vi "oa_Tachless Speed Profile Generator Popup.vi"(0 "scaled signal [EU]":waveform(dbl)={"t0"=timestamp(0 s since 1904-01-01), "dt"=0.0, "Y"=[]}) -> (3 "effective bandwidth":T3={"bandwidth value"=0.5, "bandwidth unit"=enum."Order"} {"bandwidth value" min=0.0 format="%.2f"}, 4 "dup scaled signal [EU]":waveform(dbl), 8 "speed profile":T4 {"speed [RPM]" format="%.2f"; "time [s]" format="%.2f"}, 10 "orders list":dbl[](array[numeric]) format="%.2f", 14 "window info":T5={"window type"=62, "window length"=2048} {"window type" items=["None"=0, "Hanning"=1, "Hamming"=2, "Blackman-Harris"=3, "Exact Blackman"=4, "Blackman"=5, "Flat Top"=6, "4 Term B-Harris"=7, "7 Term B-Harris"=8, "Low Sidelobe"=9, "Gaussian"=62]; "window length" min=0}, 15 "error out":errorcluster)   [LabVIEW 2017, in "SoundVib_Tachless.lvlib"]
doc: "Interactively generates speed profile from the vibration signal without tachometer signal."
uses:
  <vilib>/addons/Sound and Vibration/Order Analysis/Tachless/SoundVib_Tachless.lvlib
  <vilib>/addons/Sound and Vibration/Order Analysis/Ref Gabor Order Tracking/window information.ctl
  <vilib>/addons/Sound and Vibration/Order Analysis/Tach Process/SubVIs/speed profile.ctl
  <vilib>/addons/Sound and Vibration/Order Analysis/Ref Gabor Order Tracking/Mask Bandwidth.ctl
  <vilib>/Utility/miscctls.llb/LVPoint32TypeDef.ctl
  <vilib>/addons/Sound and Vibration/Order Analysis/Tachless/SubVIs/OAT Tachless Globa Settings.vi
  <vilib>/addons/Sound and Vibration/Order Analysis/Ref Gabor Order Tracking/Get Freq-Time Spectral Map (DBL).vi
  <vilib>/addons/Sound and Vibration/Order Analysis/_OAT State Machine/OAT State Machine Generate Event for Numeric.vi
  <vilib>/addons/Sound and Vibration/Order Analysis/Gabor Order Tracking/SoundVib_Gabor.lvlib
  <vilib>/addons/Sound and Vibration/Order Analysis/Tach Process/SoundVib_TachProcess.lvlib
panel:
  out "MouseButton":u16
  in  "symbols":i32[](array[numeric])=[8, 8, 0, 9, 9]
  in  "Items List":string[](array[string])=["Add Control Point", "Connect", "-", "Remove Control Point", "Break"]
  out "MouseCoords":T1
  out "Cursor Position":cluster{"Cursor X":dbl, "Cursor Y":dbl}
  out "XY Max Range":T2 {"YScale.Range"."Start" format="%.2f"; "YScale.Range"."Minor Incr" format="%.2f"; "YScale.Range"."Increment" format="%.2f"; "YScale.Range"."Maximum" format="%.2f"; "YScale.Range"."Minimum" format="%.2f"; "XScale.Range"."Start" format="%.2f"; "XScale.Range"."Minor Incr" format="%.2f"; "XScale.Range"."Increment" format="%.2f"; "XScale.Range"."Maximum" format="%.2f"; "XScale.Range"."Minimum" format="%.2f"}
  out "sample rate":dbl
  in  "Next":bool
  in  "Prev":bool
  in  "Cancel":bool
  in  "Update Cursor":bool
  in  "Refined Trace Color":u32(colorbox) caption="Color"
  out "new plot":bool=TRUE
  in  "Highlighted Trace Color":u32(colorbox)
  in  "Editing Trace Color":u32(colorbox)
  in  "Mask Color":u32(colorbox)
  out "ignore cursor":bool=TRUE
  in  "Popup Menu":i32(listbox)
  in  "Pop Pos":cluster{i32, i32}
  in  "chkpoint color":u32(colorbox)=16383857
  out "Tracks":cluster{"X":dbl[], "Y":dbl[]}[](graph)
  out "S&V plot":dbl[](graph)
  out "Time-Frequency Plot":dbl[][](graph)
  in  "Pos of Plot Area":bool
  in  "Tab Control":enum32{"Edit", "Refine"}(tab)
  in  "Window Length":T6(ring)=enum."512"
  in  "Current Order":dbl=1.0 format="%.2f"
  in  "Del Order":bool
  in  "Add Order":bool
  in  "Order":dbl=1.0 format="%.2f"
  in  "Reference Orders":i32[](listbox)
  in  "Show Mask":bool
  in  "Refine":bool
  in  "Bandwidth":cluster{"Mask Width":dbl, "unit":u16} {"unit" items=["Order", "Hz"]; "Mask Width" min=0.0 step=0.01 scale=0.001..1.0 scale format="%.2p"}
  # "Data"
  # "State"
  # "Mouse Popup Menu"
  # "Step 1/2 (Edit Profile)"
  # "Setting for Time-Frequency Chart"
  # "Setting for the Control Points"
  # "Tips"
  # "In this step, you should mark one certain order on the Time-Frequency Plot with control points. You can change the Window Length to make the plot clear, and edit the control points by right clicking on it. You should set the Current Order to the one you mark before going to the next step."
  # "Step 2/2 (Refine)"
  # "Setting for Refining"
  # "narrow"
  # "wide"
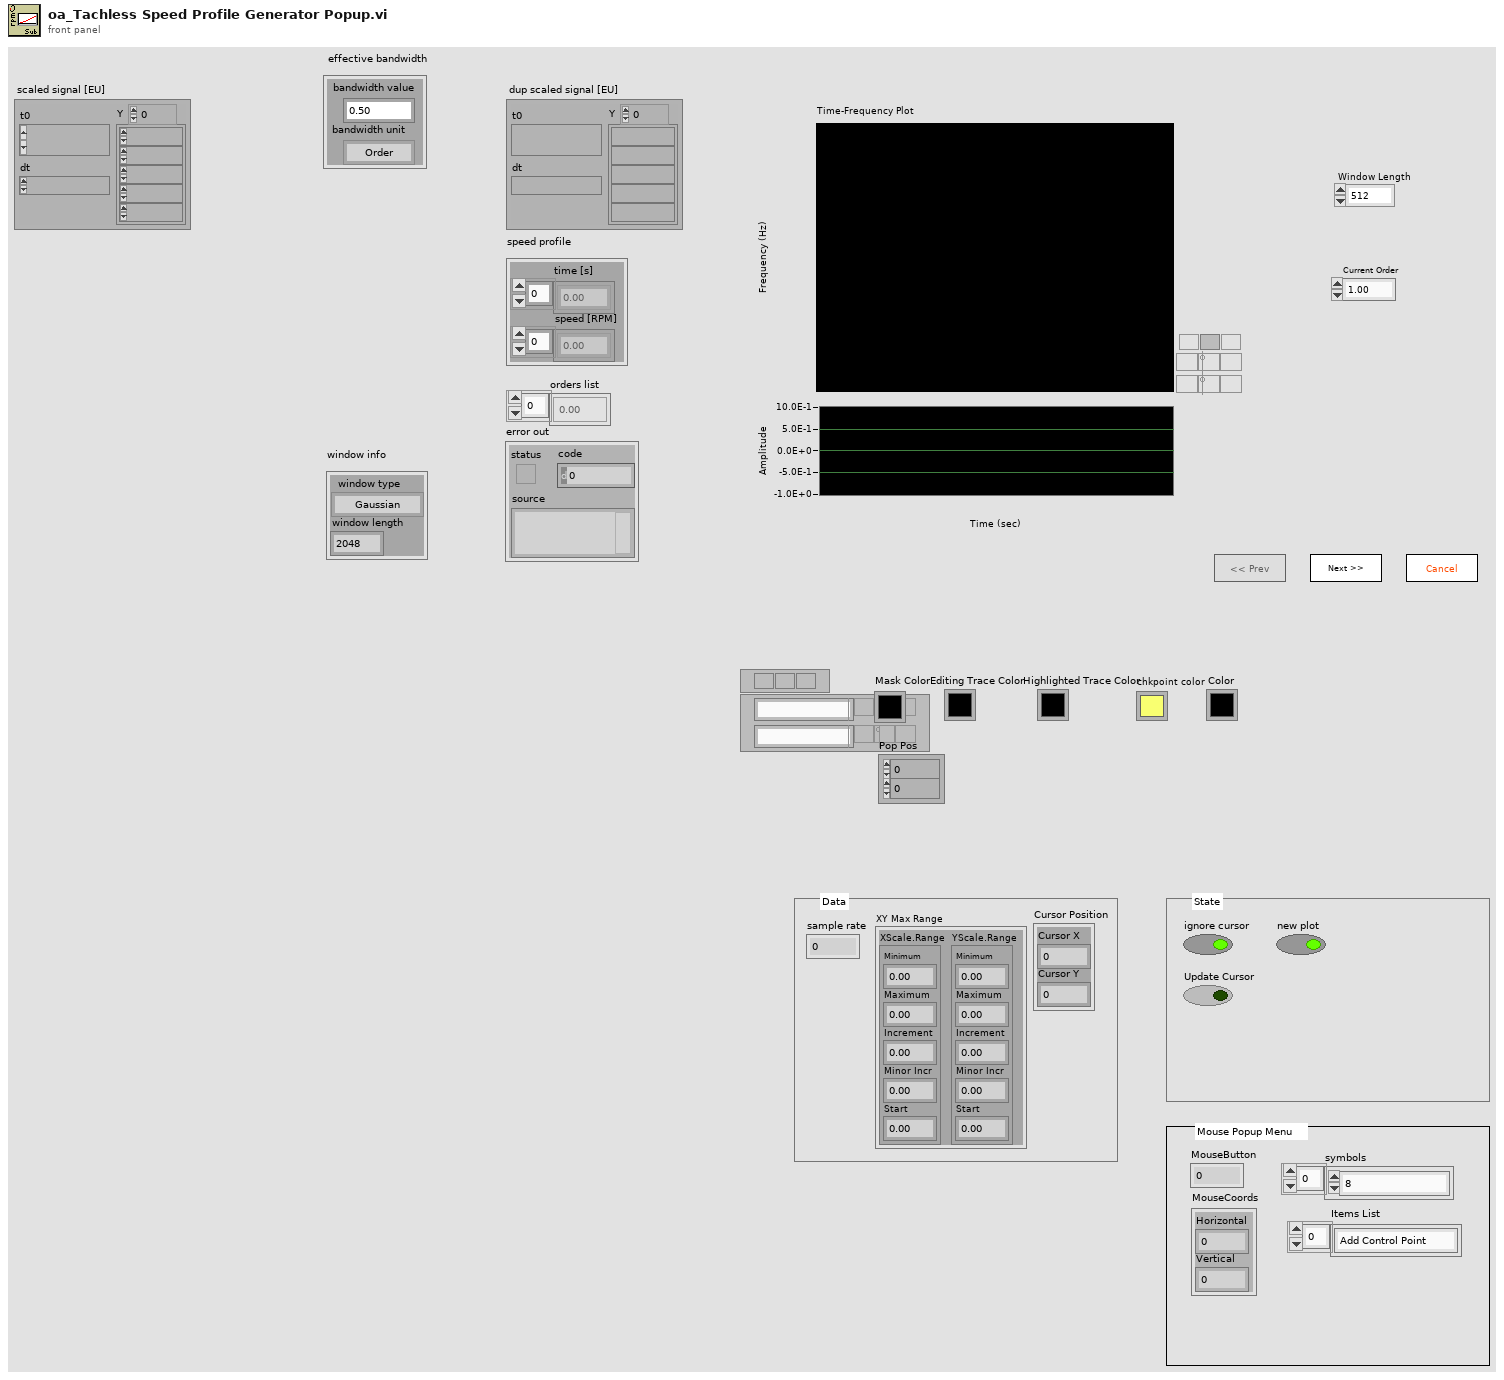
[diagram p1: front panel]
types:
  T1 = typedef "LVPoint32TypeDef.ctl" = cluster{"Horizontal":i32, "Vertical":i32}
  T2 = cluster{"XScale.Range":cluster{"Minimum":dbl, "Maximum":dbl, "Increment":dbl, "Minor Incr":dbl, "Start":dbl}, "YScale.Range":cluster{"Minimum":dbl, "Maximum":dbl, "Increment":dbl, "Minor Incr":dbl, "Start":dbl}}
  T3 = typedef "SoundVib_Gabor.lvlib/Mask Bandwidth.ctl" = cluster{"bandwidth value":dbl, "bandwidth unit":enum16{"Order", "Hz"}}
  T4 = typedef "SoundVib_TachProcess.lvlib/speed profile.ctl" = cluster{"time [s]":dbl[], "speed [RPM]":dbl[]}
  T5 = typedef "SoundVib_Gabor.lvlib/window information.ctl" = cluster{"window type":u32, "window length":i32}
  T6 = enum16{"256", "512", "1024", "2048", "4096", "8192", "16384", "32768"}
  T7 = typedef "LVPositionTypeDef.ctl" = cluster{"Left":i32, "Top":i32}
  T8 = typedef "LVBoundsTypeDef.ctl" = cluster{"Width":u32, "Height":u32}
  T9 = cluster{"Name":string, "Color":u32, "Style":u8, "Point Style":u8, "Name Visible":bool, "Allow Drag":bool, "Lock Style":u32, "Plot":u32, "Index":i32, "Position":cluster{"X":dbl, "Y":dbl}}[]
  T10 = typedef "LVPointDoubleTypeDef.ctl" = cluster{"Cursor X":dbl, "Cursor Y":dbl}
  T11 = typedef "LVRangeTypeDef.ctl" = cluster{"Minimum":dbl, "Maximum":dbl, "Increment":dbl, "Minor Increment":dbl, "Start":dbl}
  T12 = typedef "SoundVib_Gabor.lvlib/GT RefNum.ctl" = refnum<k1>
  T13 = cluster{"Cursor.Cursor X":dbl, "Cursor.Cursor X":dbl}
  T14 = cluster{"Name":string, "Color":u32, "Hair Style":u8, "Point Style":u8, "Name Visible":bool, "Trackable":bool, "Lock Style":u32, "Plot Number":u32, "Marker Index":i32, "Location":cluster{"X":dbl, "Y":dbl}}[]
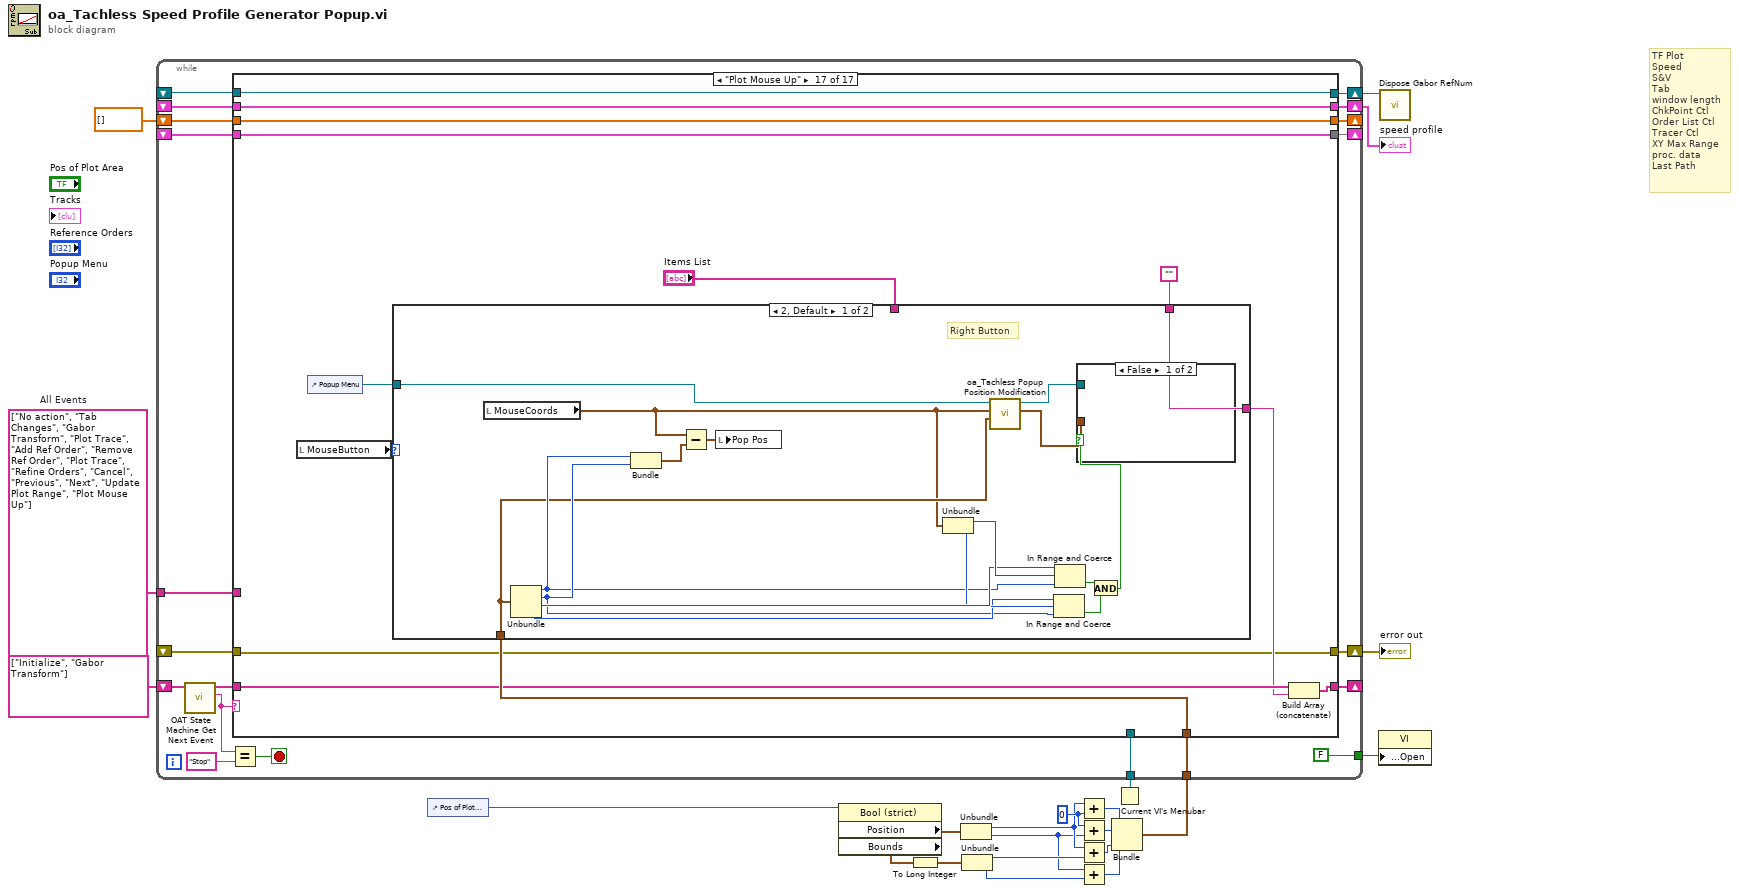
[diagram p0: block diagram]
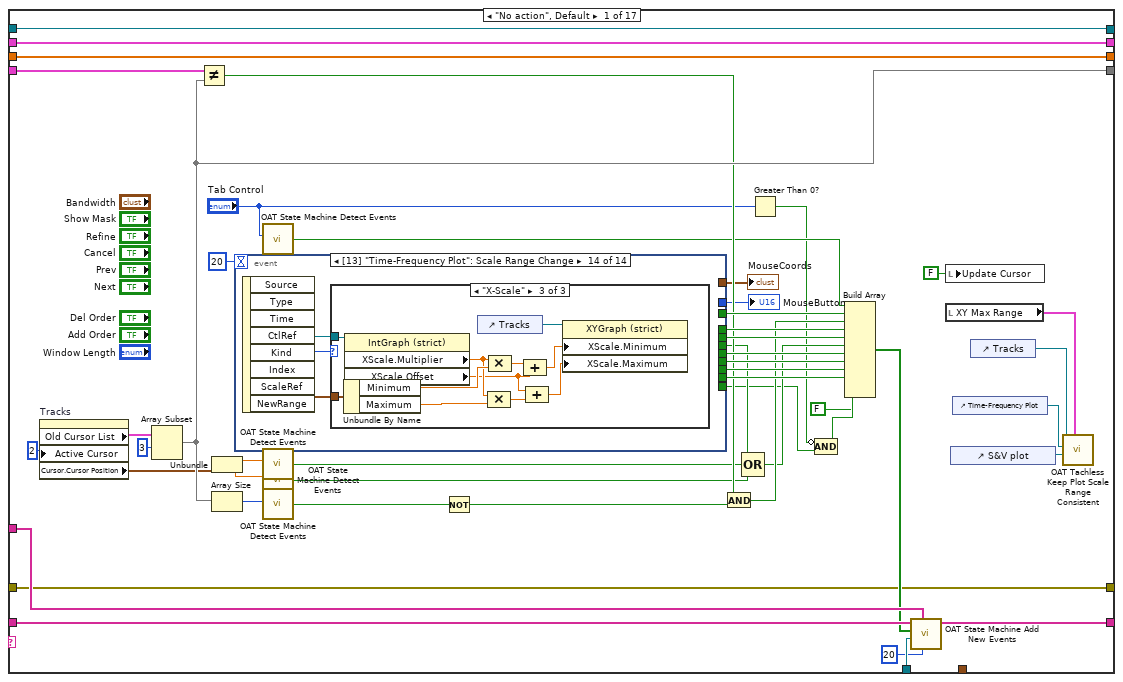
[diagram p2: hidden frame]
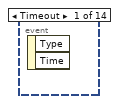
[diagram p3: hidden frame]
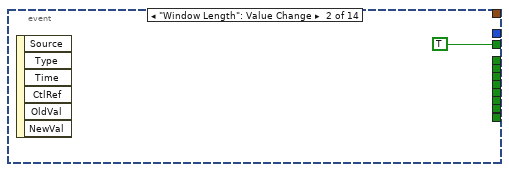
[diagram p4: hidden frame]
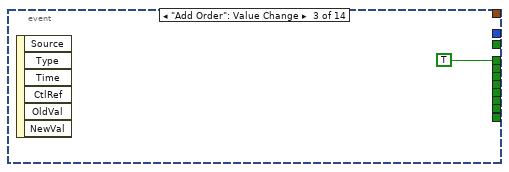
[diagram p5: hidden frame]
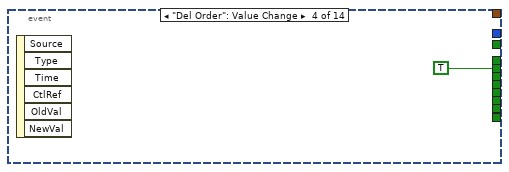
[diagram p6: hidden frame]
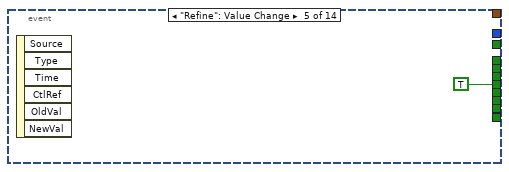
[diagram p7: hidden frame]
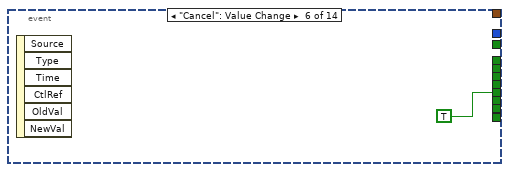
[diagram p8: hidden frame]
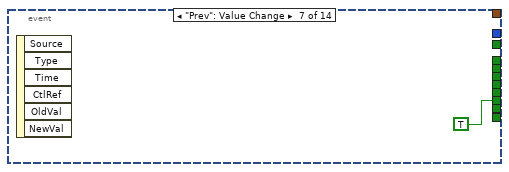
[diagram p9: hidden frame]
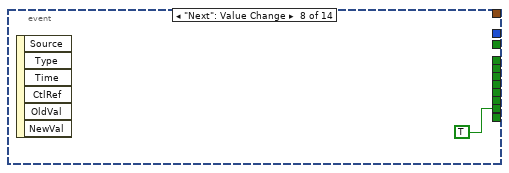
[diagram p10: hidden frame]
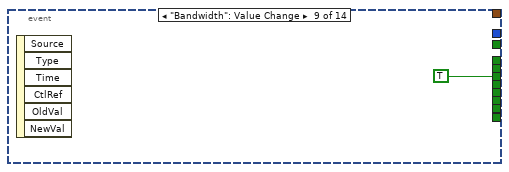
[diagram p11: hidden frame]
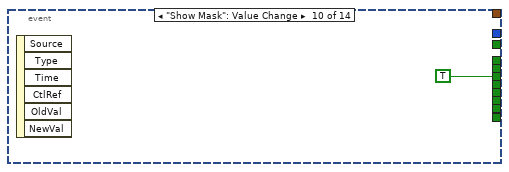
[diagram p12: hidden frame]
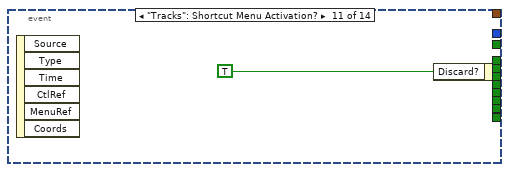
[diagram p13: hidden frame]
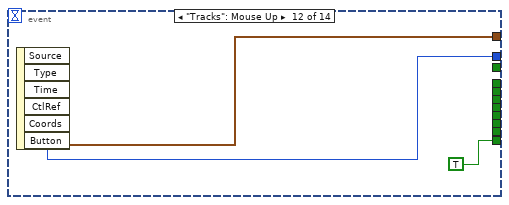
[diagram p14: hidden frame]
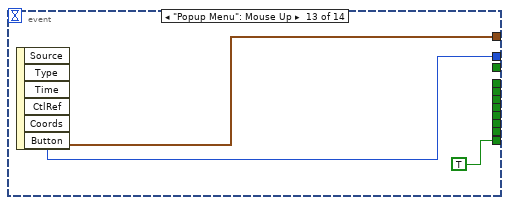
[diagram p15: hidden frame]
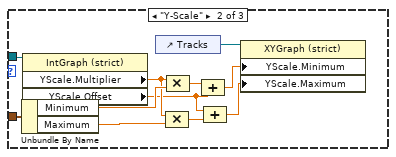
[diagram p17: hidden frame]
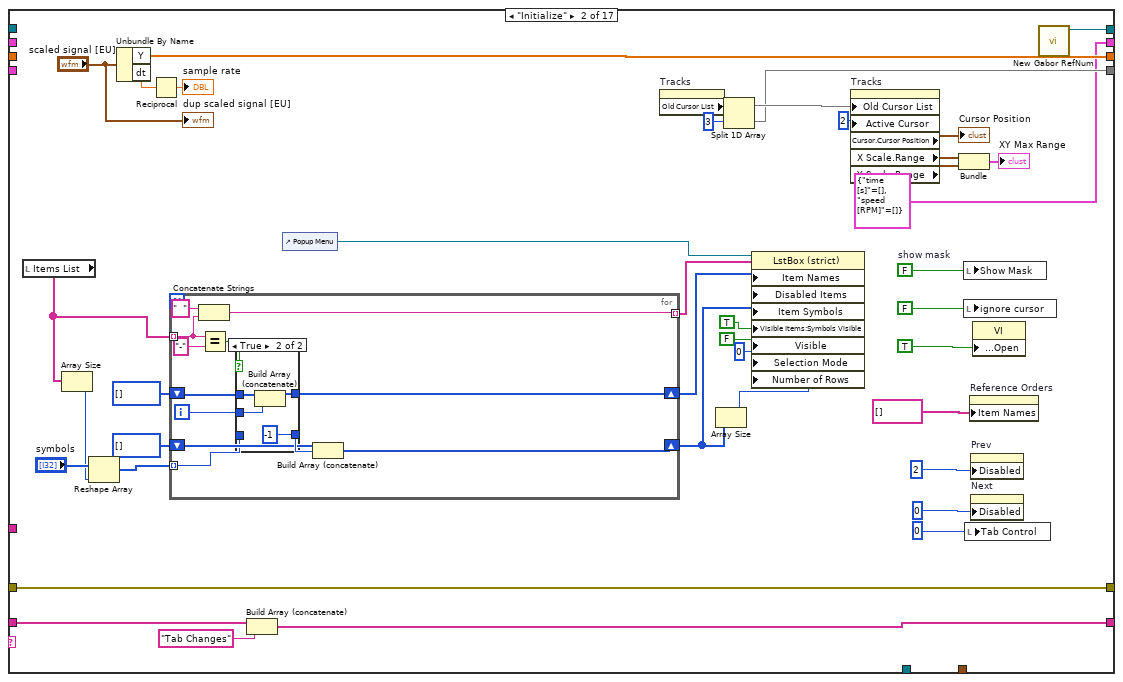
[diagram p18: hidden frame]
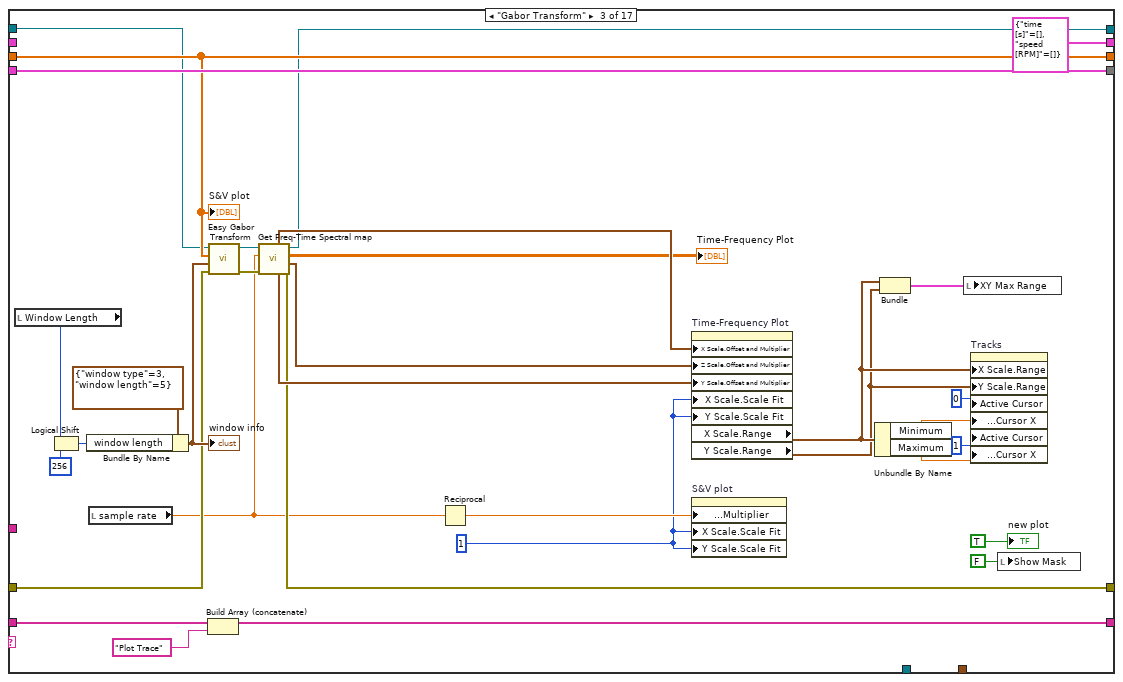
[diagram p20: hidden frame]
diagram:
  w15 = 0 ("y")
  w22 = string[] ["No action", "Tab Changes", "Gabor Transform", "Plot Trace", "Add Ref Order", "Remove Ref Order", "Plot Trace", "Refine Orders", "Cancel", "Previous", "Next", "Update Plot Range", "Plot Mouse Up"]  # All Events
  # "TF Plot\nSpeed\nS&V\nTab\nwindow length\nChkPoint Ctl\nOrder List Ctl\nTracer Ctl\nXY Max Range\nproc. data\nLast Path"
  n1 = control-ref of="Pos of Plot Area"() -> (w6:refnum<vi>)
  n2 = property on="Property Node" class="Bool (strict)"(reference=w6) -> ("Position"=w8:T7, "Bounds"=w2:T8)  [unwired: 1 in, 2 out]
  n3 = To Long Integer(number=w2) -> (32bit integer=w1:cluster{"Width":i32, "Height":i32})
  n4 = Unbundle(w8) -> ("Left"=w14:i32, "Top"=w11:i32)
  n5 = Unbundle(w1) -> ("Width"=w13:i32, "Height"=w12:i32)
  n6 = Add(x=w14, y=w15) -> (x+y=w17:i32)
  n7 = Add(x=w15, y=w11) -> (x+y=w16:i32)
  n8 = Add(x=w14, y=w13) -> (x+y=w10:i32)
  n9 = Add(x=w11, y=w12) -> (x+y=w9:i32)
  n10 = Bundle(w17, w16, w10, w9) -> (w7:cluster{i32, i32, i32, i32})  [unwired: 1 in]
  n11 = Current VI's Menubar() -> (w21:refnum<k9>)
  n12 = while {
    tunnel: w7 -> [w27]
    tunnel: w21 -> [w29]
    shift-left: _ -> [w30]
    shift-right: [w31] -> _
    tunnel: w22 -> [w36]
    shift-left: string[] ["Initialize", "Gabor Transform"] ("Event Queue Out") -> [w37]
    shift-right: [w34] -> _
    shift-left: dbl[] [] ("data") -> [w28]
    shift-right: [w38] -> _
    shift-left: _ -> [w39]
    shift-right: [w40] -> w18
    shift-left: _ -> [w41]
    shift-right: [w42] -> w20
    tunnel: [FALSE ("Front Panel Window:Open")] -> w5
    shift-right: [w24] -> w4
    shift-left: _ -> [w23]
    stop <- w26 stop-if-true
    n13 = call <vilib>:"OAT State Machine Get Next Event.vi"("event queue in"=w37) -> ("next event"=w33:string, "event queue out"=w35:string[])  [unwired: 5 in]
    n14 = Equal?(x=w33, y="Stop" ("item tag")) -> (x = y?=w26:bool)
    n15 = case shown="\"Plot Mouse Up\"" w33 {
      tunnel: [w90 w151 w206 w230 w241 w252 w263 w292 w385 w402 w412 w434 w499 w514 w523 w534 w547] -> w42
      tunnel: w41 -> [w90 _ w207 w230 w241 w252 w263 w292 w385 w402 w412 w434 w499 w514 w523 w534 w547]
      tunnel: [w89 T4 {"time [s]"=[], "speed [RPM]"=[]} ("speed profile") T4 {"time [s]"=[], "speed [RPM]"=[]} ("speed profile") w233 w244 w255 w266 w281 w368 w401 w411 w415 w500 w515 w519 w530 w546] -> w40
      tunnel: w39 -> [w89 _ _ w233 w244 w255 w266 w280 w371 w401 w411 w415 w500 w515 w519 w530 w546]
      tunnel: [w88 w162 w217 w234 w245 w256 w267 w291 w391 w400 w410 w450 w503 w517 w520 w531 w545] -> w38
      tunnel: w36 -> [w87 _ _ _ _ _ _ _ _ _ _ _ _ _ _ _ _]
      tunnel: w35 -> [w86 w171 w220 w232 w243 w254 w265 w290 w390 w399 w409 w416 w501 w510 w522 w533 w538]
      tunnel: [w48 w165 w219 w226 w239 w250 w261 w289 w383 w395 w406 w416 w501 w509 w522 w529 w537] -> w34
      tunnel: [w78 w155 w218 w231 w242 w253 w264 w275 w388 w398 w408 w435 w502 w516 w521 w532 w544] -> w31
      tunnel: w30 -> [w85 _ w218 w231 w242 w253 w264 w275 w388 w398 w408 w435 w502 w516 w521 w532 w544]
      tunnel: w29 -> [w84 _ _ _ _ _ _ _ _ _ _ _ _ _ _ _ _]
      tunnel: w28 -> [w88 _ w217 w234 w245 w256 w267 w291 w391 w400 w410 w450 w503 w517 w520 w531 w545]
      tunnel: w27 -> [_ _ _ _ _ _ _ _ _ _ _ _ _ _ _ _ w540]
      tunnel: [w59 w146 w194 w223 w235 w246 w257 w268 w347 w392 w403 w417 w496 w504 w518 w524 w535] -> w24
      tunnel: w23 -> [w59 w146 w195 w223 w235 w246 w257 w268 w347 w392 w403 w417 w496 w504 w518 w524 w535]
      frame "No action", Default {
        n16 = property on="Tracks" class="XYGraph (strict)"("Active Cursor"=u32 2) -> ("Old Cursor List"=w82:T9, "Cursor.Cursor Position"=w65:T10)  [unwired: 2 in, 2 out]
        n17 = Array Subset(array=w82, index=3) -> (w78:T9)  [unwired: 1 in]
        n18 = Not Equal?(x=w85, y=w78) -> (x != y?=w67:bool)
        n19 = Unbundle(w65) -> ("Cursor X"=w64:dbl, "Cursor Y"=w63:dbl)
        n20 = Array Size(array=w78) -> (size(s)=w77:i32)
        n21 = event shown="[13] \"Time-Frequency Plot\": Scale Range Change" {
          selector: _ -> [_ _ _ _ _ _ _ _ _ _ _ _ _ _]
          dyn-events: _ -> [_ _ _ _ _ _ _ _ _ _ _ _ _ _]
          timeout: 20 -> [_ _ _ _ _ _ _ _ _ _ _ _ _ _]
          tunnel: [_ TRUE _ _ _ _ _ _ _ _ _ _ _ _] -> w70
          tunnel: [_ _ TRUE _ _ _ _ _ _ _ _ _ _ _] -> w71
          tunnel: [_ _ _ TRUE _ _ _ _ _ _ _ _ _ _] -> w72
          tunnel: [_ _ _ _ _ _ _ _ TRUE TRUE _ _ _ _] -> w58
          tunnel: [_ _ _ _ TRUE _ _ _ _ _ _ _ _ _] -> w73
          tunnel: [_ _ _ _ _ TRUE _ _ _ _ _ _ _ _] -> w74
          tunnel: [_ _ _ _ _ _ TRUE _ _ _ _ _ _ _] -> w75
          tunnel: [_ _ _ _ _ _ _ TRUE _ _ _ _ _ _] -> w76
          tunnel: [_ _ _ _ _ _ _ _ _ _ _ TRUE TRUE _] -> w47
          tunnel: [_ _ _ _ _ _ _ _ _ _ _ w102 w106 _] -> w49
          tunnel: [_ _ _ _ _ _ _ _ _ _ _ w101 w105 _] -> w45
          event Timeout {
            n22 = event-data() -> ()  [unwired: 1 in, 2 out]
          }
          event "Window Length": Value Change {
            n23 = event-data() -> ()  [unwired: 1 in, 6 out]
          }
          event "Add Order": Value Change {
            n24 = event-data() -> ()  [unwired: 1 in, 6 out]
          }
          event "Del Order": Value Change {
            n25 = event-data() -> ()  [unwired: 1 in, 6 out]
          }
          event "Refine": Value Change {
            n26 = event-data() -> ()  [unwired: 1 in, 6 out]
          }
          event "Cancel": Value Change {
            n27 = event-data() -> ()  [unwired: 1 in, 6 out]
          }
          event "Prev": Value Change {
            n28 = event-data() -> ()  [unwired: 1 in, 6 out]
          }
          event "Next": Value Change {
            n29 = event-data() -> ()  [unwired: 1 in, 6 out]
          }
          event "Bandwidth": Value Change {
            n30 = event-data() -> ()  [unwired: 1 in, 6 out]
          }
          event "Show Mask": Value Change {
            n31 = event-data() -> ()  [unwired: 1 in, 6 out]
          }
          event "Tracks": Shortcut Menu Activation? {
            n32 = event-data() -> ()  [unwired: 1 in, 6 out]
            n33 = event-data("Discard?"=TRUE) -> ()  [unwired: 1 in, 1 out]
          }
          event "Tracks": Mouse Up {
            n34 = event-data() -> ("Coords"=w102:T1, "Button"=w101:u16)  [unwired: 1 in, 4 out]
          }
          event "Popup Menu": Mouse Up {
            n35 = event-data() -> ("Coords"=w106:T1, "Button"=w105:u16)  [unwired: 1 in, 4 out]
          }
          event "Time-Frequency Plot": Scale Range Change {
            n36 = event-data() -> ("CtlRef"=w107:refnum<vi>, "Kind"=w109:enum16{"X-Scale", "Y-Scale", "Z-Scale"}, "NewRange"=w108:T11)  [unwired: 1 in, 5 out]
            n37 = case shown="\"X-Scale\"" w109 {
              tunnel: w108 -> [_ w119 w130]
              tunnel: w107 -> [_ w120 w131]
              frame "Z-Scale", Default {
              }
              frame "Y-Scale" {
                n38 = Unbundle By Name(w119) -> ("Minimum"=w118:dbl, "Maximum"=w117:dbl)
                n39 = property class="IntGraph (strict)"(reference=w120) -> ("YScale.Multiplier"=w116:dbl, "YScale.Offset"=w113:dbl)  [unwired: 1 in, 2 out]
                n40 = control-ref of="Tracks"() -> (w112:refnum<vi>)
                n41 = Compound Arithmetic op=MULTIPLY(w116, w117) -> (w114:dbl)
                n42 = Compound Arithmetic op=MULTIPLY(w116, w118) -> (w115:dbl)
                n43 = Compound Arithmetic op=ADD(w115, w113) -> (w111:dbl)
                n44 = Compound Arithmetic op=ADD(w113, w114) -> (w110:dbl)
                n45 = property class="XYGraph (strict)"(reference=w112, "YScale.Minimum"=w111, "YScale.Maximum"=w110) -> ()  [unwired: 1 in, 2 out]
              }
              frame "X-Scale" {
                n46 = Unbundle By Name(w130) -> ("Minimum"=w129:dbl, "Maximum"=w128:dbl)
                n47 = property class="IntGraph (strict)"(reference=w131) -> ("XScale.Multiplier"=w127:dbl, "XScale.Offset"=w124:dbl)  [unwired: 1 in, 2 out]
                n48 = control-ref of="Tracks"() -> (w123:refnum<vi>)
                n49 = Compound Arithmetic op=MULTIPLY(w127, w128) -> (w125:dbl)
                n50 = Compound Arithmetic op=MULTIPLY(w127, w129) -> (w126:dbl)
                n51 = Compound Arithmetic op=ADD(w126, w124) -> (w122:dbl)
                n52 = Compound Arithmetic op=ADD(w124, w125) -> (w121:dbl)
                n53 = property class="XYGraph (strict)"(reference=w123, "XScale.Minimum"=w122, "XScale.Maximum"=w121) -> ()  [unwired: 1 in, 2 out]
              }
            }
          }
        }
        "MouseButton" <- w45
        "MouseCoords" <- w49
        n54 = call-poly <vilib>:"OAT State Machine Detect Events.vi"("Numeric"="Tab Control") -> ("Event"=w56:bool)  [unwired: 7 in]
        n55 = call-poly <vilib>:"OAT State Machine Detect Events.vi"("Numeric"=w64) -> ("Event"=w62:bool)  [unwired: 7 in]
        n56 = call-poly <vilib>:"OAT State Machine Detect Events.vi"("Numeric"=w63) -> ("Event"=w61:bool)  [unwired: 7 in]
        n57 = call-poly <vilib>:"OAT State Machine Detect Events.vi"("Numeric"=w77) -> ("Event"=w80:bool)  [unwired: 7 in]
        n58 = Not(x=w80) -> (.not. x?=w68:bool)
        n59 = And(x=w67, y=w68) -> (x .and. y?=w66:bool)
        n60 = Compound Arithmetic op=OR(w58, w62, w61) -> (w57:bool)
        n61 = Greater Than 0?(x="Tab Control") -> (x > 0?=w46:bool)
        n62 = Compound Arithmetic op=AND(invert w46, w47) -> (w44:bool)
        n63 = Build Array(w56, w70, w66, w71, w72, w57, w73, w74, w75, w76, FALSE ("element"), w44) -> (w69:bool[])
        n64 = call <vilib>:"OAT State Machine Add New Events.vi"("ms timeout (200)"=20, "Event Names"=w87, "Menu Refnum"=w84, "New Events"=w69, "Event Queue In"=w86) -> ("Event Queue Out"=w48:string[])  [unwired: 6 in]
        n65 = local write "Update Cursor"(FALSE ("Update Cursor")) -> ()
        n66 = local read "XY Max Range"() -> (w51:T2)
        n67 = control-ref of="S&V plot"() -> (w52:refnum<vi>)
        n68 = control-ref of="Time-Frequency Plot"() -> (w53:refnum<vi>)
        n69 = control-ref of="Tracks"() -> (w54:refnum<vi>)
        n70 = call <vilib>:"OAT Tachless Keep Plot Scale Range Consistent.vi"("XY Max Range"=w51, "Wavefor Plot ref"=w52, "TF Plot Ref"=w53, "Tracks Ref"=w54) -> ()  [unwired: 8 in]
      }
      frame "Initialize" {
        w166 = FALSE  # show mask
        n71 = local read "Items List"() -> (w133:string[])
        n72 = Array Size(array=w133) -> (size(s)=w134:i32)
        n73 = Reshape Array("symbols", w134) -> (w135:i32[])
        n74 = Unbundle By Name("scaled signal [EU]") -> ("Y"=w162:dbl[], "dt"=w161:dbl)
        n75 = Reciprocal(x=w161) -> (1/x=→"sample rate":dbl)
        n76 = for {
          tunnel: w133 -> [w174] mode=indexing
          shift-right: [w181] -> w144
          shift-left: i32[] [] -> [w179]
          shift-right: [w177] -> w137
          shift-left: i32[] [] -> [w176]
          tunnel: w135 -> [w175] mode=indexing
          tunnel: [w172] -> w140 mode=indexing
          i -> [w180]
          n77 = Concatenate Strings("  " ("Substring"), w174) -> (w172:string)
          n78 = Equal?(x=w174, y="-") -> (x = y?=w182:bool)
          n79 = case shown="True" w182 {
            tunnel: [w185 w189] -> w181
            tunnel: w180 -> [_ w187]
            tunnel: w179 -> [w185 w188]
            tunnel: [w184 -1] -> w178
            tunnel: w175 -> [w184 _]
            frame False {
            }
            frame True {
              n80 = Build Array (concatenate)(w188, w187) -> (w189:i32[])
            }
          }
          n81 = Build Array (concatenate)(w176, w178) -> (w177:i32[])
        }
        n82 = Build Array (concatenate)(w171, "Tab Changes") -> (w165:string[])
        n83 = control-ref of="Popup Menu"() -> (w132:refnum<vi>)
        n84 = property on="Tracks" class="XYGraph (strict)"() -> ("Old Cursor List"=w158:T9)  [unwired: 2 in, 2 out]
        n85 = Array Size(array=w137) -> (size(s)=w136:i32)
        n86 = Split 1D Array(array=w158, index=3 ("Array Length")) -> (first subarray=w156:T9, second subarray=w155:T9)
        n87 = property class="LstBox (strict)"(reference=w132, "Item Names"=w140, "Disabled Items"=w144, "Item Symbols"=w137, "Visible Items:Symbols Visible"=TRUE ("Symbols Visible"), "Visible"=FALSE, "Selection Mode"=0, "Number of Rows"=w136) -> ()  [unwired: 1 in, 2 out]
        n88 = property on="Tracks" class="XYGraph (strict)"("Old Cursor List"=w156, "Active Cursor"=u32 2) -> ("Cursor.Cursor Position"=→"Cursor Position":T10, "X Scale.Range"=w148:T11, "Y Scale.Range"=w149:T11)  [unwired: 2 in, 2 out]
        n89 = Bundle("XScale.Range"=w148, "YScale.Range"=w149) -> (→"XY Max Range":cluster{"XScale.Range":T11, "YScale.Range":T11})  [unwired: 1 in]
        n90 = local write "Show Mask"(w166) -> ()
        n91 = local write "ignore cursor"(FALSE ("ignore cursor")) -> ()
        n92 = local write "Tab Control"(0) -> ()
        n93 = property on="Reference Orders" class="LstBox (strict)"("Item Names"=string[] []) -> ()  [unwired: 2 in, 2 out]
        n94 = property on="Prev" class="Bool"("Disabled"=u8 2) -> ()  [unwired: 2 in, 2 out]
        n95 = property on="Next" class="Bool"("Disabled"=u8 0) -> ()  [unwired: 2 in, 2 out]
        n96 = property class="VI"("Front Panel Window:Open"=TRUE) -> ()  [unwired: 2 in, 2 out]
        n97 = call <vilib>:"New Gabor RefNum.vi"() -> ("RefNum"=w151:T12)  [unwired: 9 in, 1 out]
        "dup scaled signal [EU]" <- "scaled signal [EU]"
      }
      frame "Gabor Transform" {
        w211 = u8 1 ("X Scale.Scale Fit")
        n98 = local read "Window Length"() -> (w197:T6)
        n99 = Logical Shift(y=w197, x=256) -> (x << y=w213:i32)
        n100 = Bundle By Name(cluster=T5 {"window type"=3, "window length"=5} ("window information"), "window length"=w213) -> (w214:T5)
        "window info" <- w214
        n101 = local read "sample rate"() -> (w193:dbl)
        n102 = Build Array (concatenate)(w220, "Plot Trace" ("status")) -> (w219:string[])
        n103 = call <vilib>:"Easy Gabor Transform.vi"("error in (no error)"=w195, "window info"=w214, "x[n]"=w217, "RefNum in"=w207) -> ("error out"=w222:errorcluster, "RefNum out"=w221:T12)  [unwired: 3 in, 3 out]
        n104 = call-poly <vilib>:"Get Freq-Time Spectral map.vi"("error in (no error)"=w222, "sampling frequency [Hz]"=w193, "RefNum in"=w221) -> ("error out"=w194:errorcluster, "quantization info"=w208:cluster{"offset":dbl, "multiplier":dbl}, "spectral map"=→"Time-Frequency Plot":dbl[][], "RefNum out"=w206:T12, "frequency scale"=w210:cluster{"offset":dbl, "multiplier":dbl}, "time scale"=w209:cluster{"offset":dbl, "multiplier":dbl})  [unwired: 3 in]
        n105 = Reciprocal(x=w193) -> (1/x=w216:dbl)
        n106 = property on="Time-Frequency Plot" class="IntGraph (strict)"("X Scale.Offset and Multiplier"=w209, "Z Scale.Offset and Multiplier"=w208, "Y Scale.Offset and Multiplier"=w210, "X Scale.Scale Fit"=w211, "Y Scale.Scale Fit"=w211) -> ("X Scale.Range"=w192:T11, "Y Scale.Range"=w191:T11)  [unwired: 2 in, 2 out]
        n107 = property on="S&V plot" class="WFGraph (strict)"("X Scale.Offset and Multiplier:Multiplier"=w216, "X Scale.Scale Fit"=w211, "Y Scale.Scale Fit"=w211) -> ()  [unwired: 2 in, 2 out]
        n108 = Unbundle By Name(w192) -> ("Minimum"=w201:dbl, "Maximum"=w200:dbl)
        n109 = Bundle("XScale.Range"=w192, "YScale.Range"=w191) -> (w190:cluster{"XScale.Range":T11, "YScale.Range":T11})  [unwired: 1 in]
        n110 = local write "XY Max Range"(w190) -> ()
        n111 = property on="Tracks" class="XYGraph (strict)"("X Scale.Range"=w192, "Y Scale.Range"=w191, "Active Cursor"=u32 0, "Cursor.Cursor Position:Cursor X"=w201, "Active Cursor"=u32 1, "Cursor.Cursor Position:Cursor X"=w200) -> ()  [unwired: 2 in, 2 out]
        n112 = local write "Show Mask"(FALSE ("Show Mask")) -> ()
        "S&V plot" <- w217
        "new plot" <- TRUE
      }
      frame "Add Control Point" {
        n113 = Build Array (concatenate)(w232, "Plot Trace") -> (w226:string[])
        n114 = control-ref of="Tracks"() -> (w227:refnum<vi>)
        n115 = local write "Update Cursor"(TRUE ("Update Cursor")) -> ()
        n116 = call <vilib>:"OAT Tachless Add Control Point.vi"("chkpoint color"="chkpoint color", "Pop Pos"="Pop Pos", "Tracks Ref"=w227) -> ()  [unwired: 9 in]
      }
      frame "Remove Control Point" {
        n117 = Build Array (concatenate)(w243, "Plot Trace") -> (w239:string[])
        n118 = local read "Pop Pos"() -> (w237:cluster{i32, i32})
        n119 = control-ref of="Tracks"() -> (w240:refnum<vi>)
        n120 = local write "Update Cursor"(TRUE ("Update Cursor")) -> ()
        n121 = call <vilib>:"OAT Tachless Remove Control Point.vi"("Pop Pos"=w237, "Tracks Ref"=w240) -> ()  [unwired: 10 in]
      }
      frame "Break" {
        n122 = Build Array (concatenate)(w254, "Plot Trace") -> (w250:string[])
        n123 = local read "Pop Pos"() -> (w248:cluster{i32, i32})
        n124 = control-ref of="Tracks"() -> (w251:refnum<vi>)
        n125 = call <vilib>:"OAT Tachless Break Trace.vi"("Pop Pos"=w248, "Tracks Ref"=w251) -> ()  [unwired: 10 in]
        n126 = local write "Update Cursor"(TRUE ("Update Cursor")) -> ()
      }
      frame "Connect" {
        n127 = Build Array (concatenate)(w265, "Plot Trace") -> (w261:string[])
        n128 = local read "Pop Pos"() -> (w259:cluster{i32, i32})
        n129 = control-ref of="Tracks"() -> (w262:refnum<vi>)
        n130 = local write "Update Cursor"(TRUE ("Update Cursor")) -> ()
        n131 = call <vilib>:"OAT Tachless Connect Trace.vi"("Pop Pos"=w259, "Tracks Ref"=w262) -> ()  [unwired: 10 in]
      }
      frame "Tab Changes" {
        n132 = local read "Window Length"() -> (w274:T6)
        n133 = local read "Tab Control"() -> (w270:enum32{"Edit", "Refine"})
        n134 = local read "XY Max Range"() -> (w269:T2)
        n135 = case shown="\"Refine\", Default" w270 {
          tunnel: w290 -> [w320 w344]
          tunnel: [w321 w343] -> w289
          tunnel: [FALSE ("Cursor.Visible") TRUE ("Cursor.Visible")] -> w284
          tunnel: [TRUE ("Cursor.Visible") FALSE ("Cursor.Visible")] -> w282
          tunnel: w269 -> [w317 _]
          tunnel: [w316 w341] -> w281
          tunnel: w280 -> [w307 w341]
          tunnel: w274 -> [w314 _]
          tunnel: ["Highlighted Trace Color" u32 16777216] -> w277
          tunnel: [u32 16777216 "Editing Trace Color"] -> w276
          tunnel: [u8 2 ("Disabled") u8 0 ("Disabled")] -> w273
          tunnel: ["Finish" ("Boolean Text.Text") "Next >>" ("Boolean Text.Text")] -> w272
          tunnel: [u8 0 ("Disabled") u8 2 ("Disabled")] -> w271
          frame "Refine", Default {
            n136 = local read "Current Order"() -> (w303:dbl)
            n137 = local read "new plot"() -> (w310:bool)
            n138 = control-ref of="Time-Frequency Plot"() -> (w318:refnum<vi>)
            n139 = control-ref of="Tracks"() -> (w319:refnum<vi>)
            n140 = local write "Show Mask"(TRUE ("Show Mask")) -> ()
            n141 = Number To Fractional String(number=w303, precision (6)=i16 2) -> (F-format string=w302:string)  [unwired: 2 in]
            n142 = Build Array(w302) -> (w301:string[])
            n143 = Unbundle(w307) -> ("speed [RPM]"=w306:dbl[])  [unwired: 1 out]
            n144 = property on="Reference Orders" class="LstBox (strict)"("Item Names"=w301) -> ()  [unwired: 2 in, 2 out]
            n145 = Array Max & Min(array=w306) -> (max value=w305:dbl)  [unwired: 3 out]
            n146 = property on="Tracks" class="XYGraph (strict)"("Active Cursor"=u32 2, "Cursor.Cursor Position:Cursor Y"=w305) -> ()  [unwired: 2 in, 2 out]
            n147 = Build Array (concatenate)(w320, "Plot Trace" ("status")) -> (w321:string[])
            n148 = call <vilib>:"OAT Tachless Get Speed from Chkpoint.vi"("chkpoint order"=w303, "XY Max Range"=w317, "TF Plot Ref"=w318, "Tracks ref"=w319) -> ("Current min RPM"=w313:dbl, "speed profile"=w316:T4)  [unwired: 5 in, 1 out]
            n149 = case shown="True" w310 {
              tunnel: w314 -> [_ w329]
              tunnel: w313 -> [_ w328]
              tunnel: [FALSE FALSE] -> w309
              frame False {
              }
              frame True {
                n150 = global read "OAT Tachless Globa Settings.vi" "Default Mask \nWidth (Pixels)"() -> (w330:i32)
                n151 = local read "sample rate"() -> (w325:dbl)
                n152 = call <vilib>:"OAT Tachless Get Default Refine Bandwidth.vi"("min RPM"=w328, "Window Length"=w329, "Default Mask \nWidth (Pixels)"=w330, "Sample Rate (Hz)"=w325) -> ("bandwidth"=w327:T3)  [unwired: 7 in]
                n153 = local write "Bandwidth"(w327) -> ()
              }
            }
            n154 = local write "new plot"(w309) -> ()
          }
          frame "Edit" {
            n155 = local read "Tracks"() -> (w337:cluster{"X":dbl[], "Y":dbl[]}[])
            n156 = local write "Show Mask"(FALSE ("Show Mask")) -> ()
            n157 = Replace Array Subset(array=w337, new element=cluster{"X":dbl[], "Y":dbl[]} {"X"=[], "Y"=[]} ("New Element/Subarray"), index=1 ("Index")) -> (w338:cluster{"X":dbl[], "Y":dbl[]}[])
            n158 = Build Array (concatenate)(w344, "Plot Trace") -> (w343:string[])
            n159 = local write "Tracks"(w338) -> ()
          }
        }
        n160 = property on="Tracks" class="XYGraph (strict)"() -> ("Old Cursor List"=w285:T9)  [unwired: 2 in, 2 out]
        n161 = Array Size(array=w285) -> (size(s)=w286:i32)
        n162 = property on="Next" class="Bool"("Disabled"=w273, "Boolean Text.Text"=w272) -> ()  [unwired: 2 in, 2 out]
        n163 = Subtract(x=w286, y=3) -> (x-y=w288:i32)
        n164 = for {
          N: w288 -> [_]
          tunnel: w284 -> [w293]
          i -> [w296]
          n165 = Add(x=3, y=w296) -> (x+y=w295:i32)
          n166 = property on="Tracks" class="XYGraph (strict)"("Active Cursor"=w295, "Cursor.Visible"=w293) -> ()  [unwired: 2 in, 2 out]
        }
        n167 = property on="Tracks" class="XYGraph (strict)"("Active Cursor"=u32 2, "Cursor.Visible"=w282) -> ()  [unwired: 2 in, 2 out]
        n168 = property on="Tracks" class="XYGraph (strict)"("Active Plot"=0, "Plot.Plot Color"=w276, "Active Plot"=1, "Plot.Plot Color"=w277) -> ()  [unwired: 2 in, 2 out]
        n169 = property on="Prev" class="Bool"("Disabled"=w271) -> ()  [unwired: 2 in, 2 out]
      }
      frame "Refine Orders" {
        n170 = property on="Tracks" class="XYGraph (strict)"() -> ("Old Cursor List"=w378:T9)  [unwired: 2 in, 2 out]
        n171 = local read "Bandwidth"() -> (w348:cluster{"Mask Width":dbl, "unit":u16})
        "effective bandwidth" <- w348
        n172 = local read "sample rate"() -> (w349:dbl)
        n173 = property on="Reference Orders" class="LstBox (strict)"() -> ("Item Names"=w389:string[])  [unwired: 2 in, 2 out]
        n174 = property on="Next" class="Bool"("Disabled"=u8 0) -> ()  [unwired: 2 in, 2 out]
        n175 = property on="Tracks" class="XYGraph (strict)"("Active Cursor"=u32 0 ("Write Attribute"), "Active Cursor"=u32 1 ("Write Attribute")) -> ("Cursor.Cursor Position:Cursor X"=w363:dbl, "Cursor.Cursor Position:Cursor X"=w362:dbl)  [unwired: 2 in, 2 out]
        n176 = control-ref of="Time-Frequency Plot"() -> (w380:refnum<vi>)
        n177 = Fract/Exp String To Number(string=w389) -> (number=w384:dbl[])  [unwired: 3 in, 1 out]
        n178 = Add(x=w363, y=w362) -> (x+y=w361:dbl)
        n179 = Bundle("Cursor.Cursor X"=w363, "Cursor.Cursor X"=w362) -> (w381:T13)  [unwired: 1 in]
        n180 = Split 1D Array(array=w378, index=3) -> (first subarray=w375:T9, second subarray=w379:T9)
        n181 = Scale By Power Of 2(n=-1, x=w361) -> (x*2^n=w352:dbl)
        n182 = call <vilib>:"OAT Tachless Refine Speed Profile.vi"("TF Plot Ref"=w380, "Chkpnt Order"="Current Order", "Time Boundary"=w381, "sampling frequency [Hz]"=w349, "bandwidth"=w348, "interested orders list"=w384, "refined profile"=w371, "RefNum"=w385) -> ("refined profile"=w368:T4)  [unwired: 3 in]
        n183 = Build Array (concatenate)(w390, "Plot Trace") -> (w383:string[])
        n184 = call <vilib>:"OAT Tachless Update Cursor After Refine.vi"("refined profile"=w368, "Chkpnt Order"="Current Order", "cursors"=w379) -> ("cursors out"=w376:T14)  [unwired: 8 in]
        n185 = Unbundle(w368) -> ("time [s]"=w358:dbl[], "speed [RPM]"=w367:dbl[])
        n186 = Threshold 1D Array(2:w352, 3:w358) -> (0:w357:dbl)  [unwired: 1 in]
        n187 = Divide(x=w367, y=60.0) -> (x/y=w356:dbl[])
        n188 = Build Array (concatenate)(w375, w376) -> (w350:T14)
        n189 = Interpolate 1D Array(1:w357, 2:w356) -> (0:w355:dbl)
        n190 = local read "Tracks"() -> (w370:cluster{"X":dbl[], "Y":dbl[]}[])
        n191 = Bundle("time [s]"=w358, w356) -> (w365:cluster{"time [s]":dbl[], dbl[]})  [unwired: 1 in]
        n192 = Multiply(x=w355, y="Current Order") -> (x*y=w353:dbl)
        n193 = Bundle(w352, w353) -> (w351:cluster{dbl, dbl})  [unwired: 1 in]
        n194 = local write "Show Mask"(FALSE ("Show Mask")) -> ()
        n195 = Replace Array Subset(array=w370, new element=w365, index=1 ("Index")) -> (w374:cluster{"X":dbl[], "Y":dbl[]}[])
        n196 = property on="Tracks" class="XYGraph (strict)"("Old Cursor List"=w350, "Active Cursor"=u32 2, "Cursor.Cursor Position"=w351) -> ()  [unwired: 2 in, 2 out]
        n197 = local write "Tracks"(w374) -> ()
        "ignore cursor" <- TRUE
      }
      frame "Add Ref Order" {
        n198 = control-ref of="Reference Orders"() -> (w397:refnum<vi>)
        n199 = call <vilib>:"OAT Tachless Add Del Order List.vi"("Order"="Order", "List Ctl"=cluster{"Add":bool, "Del":bool} {"Add"=TRUE, "Del"=FALSE}, "Order List ref"=w397) -> ()  [unwired: 9 in]
        n200 = Build Array (concatenate)(w399, "Plot Trace") -> (w395:string[])
      }
      frame "Remove Ref Order" {
        n201 = control-ref of="Reference Orders"() -> (w407:refnum<vi>)
        n202 = call <vilib>:"OAT Tachless Add Del Order List.vi"("List Ctl"=cluster{"Add":bool, "Del":bool} {"Add"=FALSE, "Del"=TRUE}, "Order List ref"=w407) -> ()  [unwired: 10 in]
        n203 = Build Array (concatenate)(w409, "Plot Trace") -> (w406:string[])
      }
      frame "Plot Trace" {
        n204 = local read "Show Mask"() -> (w418:bool)
        n205 = local read "XY Max Range"() -> (w420:T2)
        n206 = local read "Bandwidth"() -> (w419:cluster{"Mask Width":dbl, "unit":u16})
        n207 = local read "sample rate"() -> (w421:dbl)
        n208 = local read "Current Order"() -> (w422:dbl)
        n209 = property on="Reference Orders" class="LstBox (strict)"() -> ("Item Names"=w449:string[])  [unwired: 2 in, 2 out]
        n210 = property on="Tracks" class="XYGraph (strict)"("Active Cursor"=u32 2) -> ("Cursor.Cursor Position"=w413:T10)  [unwired: 2 in, 2 out]
        n211 = property on="Tracks" class="XYGraph (strict)"("Active Cursor"=u32 0 ("Write Attribute"), "Active Cursor"=u32 1 ("Write Attribute")) -> ("Cursor.Cursor Position:Cursor X"=w441:dbl, "Cursor.Cursor Position:Cursor X"=w440:dbl)  [unwired: 2 in, 2 out]
        n212 = control-ref of="Tracks"() -> (w437:refnum<vi>)
        n213 = Fract/Exp String To Number(string=w449) -> (number=w448:dbl[])  [unwired: 3 in, 1 out]
        "orders list" <- w448
        n214 = call <vilib>:"OAT Tachless Update Chkpoints (Auto Place).vi"("Update Cursor"="Update Cursor", "RefNum"=w434, "sampling frequency [Hz]"=w421, "XY Max Range"=w420, "Tracks ref"=w437) -> ("Boundary"=w436:cluster{"X":dbl[], "Y":dbl[]}, "ChkPoints"=w431:cluster{"X":dbl[], "Y":dbl[]})  [unwired: 5 in]
        n215 = call <vilib>:"OAT Tachless Get Order Profile at Cursor.vi"("Cursor Position"=w413, "speed profile"=w415) -> ("order at cursor"=w423:dbl, "Profile at Cursor"=w424:cluster{"time [s]":dbl[], dbl[]})  [unwired: 8 in]
        n216 = local read "Tab Control"() -> (w426:enum32{"Edit", "Refine"})
        n217 = local write "ignore cursor"("Update Cursor") -> ()
        n218 = Bundle("Cursor.Cursor X"=w441, "Cursor.Cursor X"=w440) -> (w439:T13)  [unwired: 1 in]
        n219 = Not(x=w418) -> (.not. x?=w429:bool)
        n220 = Greater Than 0?(x=w426) -> (x > 0?=w425:bool)
        n221 = And(x=w429, y=w425) -> (x .and. y?=w430:bool)
        n222 = case shown="True" w418 {
          tunnel: w448 -> [_ w465]
          tunnel: w419 -> [_ w464]
          tunnel: [w457 w463] -> w446
          tunnel: w415 -> [_ w462]
          tunnel: w439 -> [_ w461]
          tunnel: [w457 w459] -> w438
          tunnel: [w456 cluster{"time [s]":dbl[], dbl[]} {"time [s]"=[], []}] -> w428
          tunnel: w424 -> [w456 _]
          frame False {
            w457 = cluster{"time [s]":dbl[], "limit [Hz]":dbl[]}[] []
          }
          frame True {
            n223 = call <vilib>:"OAT Tachless Limit of Mask Orders.vi"("Time Boundary"=w461, "bandwidth"=w464, "reference orders"=w465, "speed profile"=w462) -> ("lower limits"=w463:cluster{"time [s]":dbl[], "limit [Hz]":dbl[]}[], "upper limits"=w460:cluster{"time [s]":dbl[], "limit [Hz]":dbl[]}[])  [unwired: 6 in]
            n224 = Interleave 1D Arrays(w460, w463) -> (w459:cluster{"time [s]":dbl[], "limit [Hz]":dbl[]}[])
          }
        }
        n225 = case shown="True" w430 {
          tunnel: w448 -> [_ w455]
          tunnel: w415 -> [_ w454]
          tunnel: [cluster{"X":dbl[], "Y":dbl[]}[] [] ("interested orders") w453] -> w433
          tunnel: w422 -> [_ w452]
          frame False {
          }
          frame True {
            n226 = call <vilib>:"OAT Tachless Band Limit of Chkpoints.vi"("interested orders list"=w455, "Current Order"=w452, "speed profile"=w454) -> ("interested orders"=w453:cluster{"X":dbl[], "Y":dbl[]}[])  [unwired: 6 in, 2 out]
          }
        }
        n227 = Build Array (concatenate)(w431, w428, w436, w438, w433) -> (w447:cluster{"X":dbl[], "Y":dbl[]}[])
        n228 = Array Size(array=w446) -> (size(s)=w445:i32)
        n229 = Array Size(array=w433) -> (size(s)=w432:i32)
        n230 = stacked-sequence {
          tunnel: w447 -> [w466 _ _ _ _]
          tunnel: "Mask Color" -> [_ _ w469 _ _]
          tunnel: w445 -> [_ _ w468 w479 _]
          tunnel: w432 -> [_ _ _ w480 _]
          tunnel: w423 -> [_ _ _ _ w494]
          tunnel: w430 -> [_ _ _ _ w488]
          frame #0 {
            n231 = local write "Tracks"(w466) -> ()
          }
          frame #1 {
            n232 = Wait (ms)(milliseconds to wait=u32 100) -> ()  [unwired: 1 out]
          }
          frame #2 {
            n233 = for {
              N: w468 -> [_]
              tunnel: w469 -> [w470]
              i -> [w476]
              n234 = Multiply(x=2, y=w476) -> (x*y=w474:i32)
              n235 = Add(x=4, y=w474) -> (x+y=w472:i32)
              n236 = Decrement(x=w472) -> (x-1=w471:i32)
              n237 = property on="Tracks" class="XYGraph (strict)"("Active Plot"=w472, "Plot.Plot Color"=w470, "Plot.Fill To"=w471, "Plot.Fill/Point Color"=w470, "Active Plot"=w471, "Plot.Plot Color"=w470) -> ()  [unwired: 2 in, 2 out]
            }
          }
          frame #3 {
            n238 = Multiply(x=2, y=w479) -> (x*y=w478:i32)
            n239 = for {
              N: w480 -> [_]
              tunnel: w478 -> [w484]
              i -> [w483]
              n240 = Compound Arithmetic op=ADD(w484, 3 ("x"), w483) -> (w485:i32)
              n241 = property on="Tracks" class="XYGraph (strict)"("Active Plot"=w485, "Plot.Plot Color"="Refined Trace Color", "Plot.Fill To"=i16 -1) -> ()  [unwired: 2 in, 2 out]
            }
          }
          frame #4 {
            n242 = Multiply(x=w494, y=60.0) -> (x*y=w490:dbl)
            n243 = Format Into String(format string="%.2f" ("Format String"), initial string=" Order " ("Input String"), w490) -> (resulting string=w487:string)  [unwired: 1 in, 1 out]
            n244 = property on="Tracks" class="XYGraph (strict)"("Active Cursor"=u32 2, "Cursor.Cursor Name"=w487, "Cursor.Cursor Name Visible"=TRUE, "Cursor.Visible"=w488) -> ()  [unwired: 2 in, 2 out]
          }
        }
      }
      frame "Previous" {
        n245 = local read "Tab Control"() -> (w498:enum32{"Edit", "Refine"})
        n246 = Decrement(x=w498) -> (x-1=w497:enum32{"Edit", "Refine"})
        n247 = local write "Tab Control"(w497) -> ()
      }
      frame "Next" {
        n248 = local read "Tab Control"() -> (w512:enum32{"Edit", "Refine"})
        n249 = Equal?(x=w512, y=enum32{"Edit", "Refine"}."Refine" ("Tab Control")) -> (x = y?=w508:bool)
        n250 = Increment(x=w512) -> (x+1=w513:enum32{"Edit", "Refine"})
        n251 = Select(t="Stop" ("status"), s=w508, f="") -> (s? t:f=w505:string)
        n252 = local write "Tab Control"(w513) -> ()
        n253 = Build Array (concatenate)(w510, w505) -> (w509:string[])
      }
      frame "Stop" {
      }
      frame "Cancel" {
        n254 = Build Array (concatenate)(w533, "Stop" ("item tag")) -> (w529:string[])
        n255 = Current VI's Path() -> (path=w527:path)
        n256 = Strip Path(path=w527) -> (name=w526:string)  [unwired: 1 out]
        n257 = Bundle(cluster=errorcluster {"status"=TRUE, "code"=43, "source"=""} ("error in (no error)"), "source"=w526) -> ()  [unwired: 2 in, 1 out]
      }
      frame "Plot Mouse Up" {
        n258 = local read "MouseButton"() -> (w539:u16)
        n259 = control-ref of="Popup Menu"() -> (w541:refnum<vi>)
        n260 = case shown="2, Default" w539 {
          tunnel: "Items List" -> [_ w574]
          tunnel: [w554 w573] -> w536
          tunnel: "" ("String") -> [w554 w569]
          tunnel: w541 -> [w551 w572]
          tunnel: w540 -> [w550 _]
          frame 2, Default {
            # "Right Button"
            n261 = local read "MouseCoords"() -> (w549:T1)
            n262 = Unbundle(w550) -> (w555:i32, w557:i32, w563:i32, w561:i32)
            n263 = Bundle(w555, w557) -> (w556:cluster{i32, i32})  [unwired: 1 in]
            n264 = Subtract(x=w549, y=w556) -> (x-y=w548:T1)
            n265 = local write "Pop Pos"(w548) -> ()
            n266 = Unbundle(w549) -> ("Horizontal"=w564:i32, "Vertical"=w562:i32)
            n267 = call <vilib>:"oa_Tachless Popup Position Modification.vi"("Pop Area"=w550, "mouse position"=w549, "Popup Menu"=w551) -> ("position"=w552:cluster{i32, i32}, "dup Popup Menu"=w553:refnum<vi>)  [unwired: 7 in]
            n268 = In Range and Coerce(upper limit=w561, x=w562, lower limit=w557) -> (In Range?=w559:bool)  [unwired: 1 out]
            n269 = In Range and Coerce(upper limit=w563, x=w564, lower limit=w555) -> (In Range?=w560:bool)  [unwired: 1 out]
            n270 = And(x=w560, y=w559) -> (x .and. y?=w558:bool)
            n271 = case shown="False" w558 {
              tunnel: w553 -> [_ w568]
              tunnel: w552 -> [_ w565]
              frame False {
              }
              frame True {
                n272 = property class="LstBox (strict)"(reference=w568, "Visible"=TRUE, "Position"=w565, "Value"=-1) -> ()  [unwired: 1 in, 2 out]
              }
            }
          }
          frame 1 {
            # "Left Button"
            n273 = property class="LstBox (strict)"(reference=w572) -> (reference out=w570:refnum<vi>, "Visible"=w571:bool)  [unwired: 1 in, 1 out]
            n274 = case shown="True" w571 {
              tunnel: w574 -> [_ w578]
              tunnel: [w575 w577] -> w573
              tunnel: w570 -> [_ w576]
              tunnel: w569 -> [w575 _]
              frame False {
              }
              frame True {
                n275 = property class="LstBox (strict)"(reference=w576, "Visible"=FALSE) -> ("Value"=w579:i32)  [unwired: 1 in, 2 out]
                n276 = Index Array(array=w578, index=w579) -> (element=w577:string)
              }
            }
          }
        }
        n277 = Build Array (concatenate)(w538, w536) -> (w537:string[])
      }
    }
  }
  "speed profile" <- w18
  "error out" <- w4
  n278 = property class="VI"("Front Panel Window:Open"=w5) -> ()  [unwired: 2 in, 2 out]
  n279 = call <vilib>:"Dispose Gabor RefNum.vi"("RefNum in"=w20) -> ()  [unwired: 7 in, 1 out]
